vi "oa_Adjust DC Gap Data for Probe Orientation.vi"(6 "rotating settings":T1={"shaft rotating direction"=0, "probe orientation"={"X (red)"=0, "Y (blue)"=90}} {"shaft rotating direction" items=["CCW", "CW"]}, 8 "error in (no error)":errorcluster, 11 "DC Gap":cluster{"X":dbl[], "Y":dbl[]}[](array[cluster]) {"Y" format="%.2f"; "X" format="%.2f"}) -> (0 "error out":errorcluster, 3 "DC Gap out":cluster{"X":dbl[], "Y":dbl[]}[](array[cluster]) {"Y" format="%.2f"; "X" format="%.2f"})   [LabVIEW 2017]
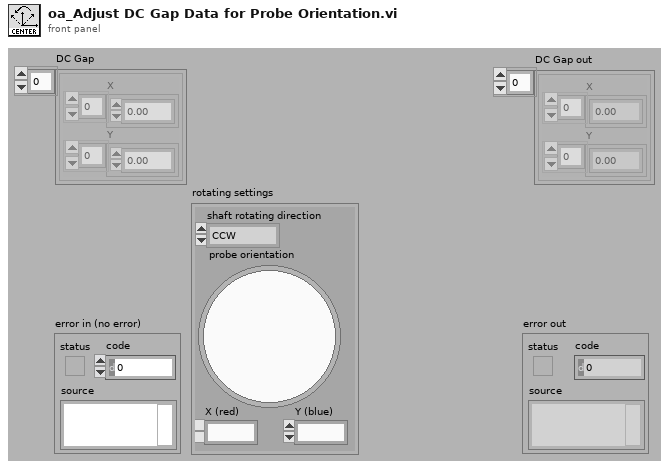
[diagram p1: front panel]
types:
  T1 = cluster{"shaft rotating direction":u16, "probe orientation":cluster{"X (red)":u32, "Y (blue)":u32}}
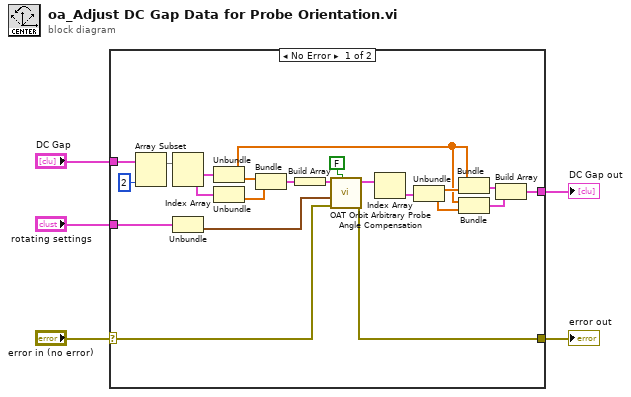
[diagram p0: block diagram]
diagram:
  n1 = case shown="No Error" "error in (no error)" {
    selector: "error in (no error)" -> [w25 w29]
    tunnel: [w23 w29] -> w4
    tunnel: "rotating settings" -> [w27 _]
    tunnel: [w6 w28] -> w2
    tunnel: "DC Gap" -> [w18 w28]
    frame No Error {
      n2 = Array Subset(array=w18, length=2) -> (w17:cluster{"X":dbl[], "Y":dbl[]}[])  [unwired: 1 in]
      n3 = Index Array(array=w17) -> (element #1=w22:cluster{"X":dbl[], "Y":dbl[]}, element #2=w21:cluster{"X":dbl[], "Y":dbl[]})  [unwired: 2 in]
      n4 = Unbundle(w27) -> ("probe orientation"=w26:cluster{"X (red)":u32, "Y (blue)":u32})  [unwired: 1 out]
      n5 = Unbundle(w22) -> ("X"=w10:dbl[], "Y"=w20:dbl[])
      n6 = Unbundle(w21) -> ("Y"=w19:dbl[])  [unwired: 1 out]
      n7 = Bundle("Y"=w20, "Y"=w19) -> (w15:cluster{"Y":dbl[], "Y":dbl[]})  [unwired: 1 in]
      n8 = Build Array(w15) -> (w14:cluster{"Y":dbl[], "Y":dbl[]}[])
      n9 = call <vilib>:"OAT Orbit Arbitrary Probe Angle Compensation.vi"("select methods"=FALSE, "error in (no error)"=w25, "probe angle"=w26, "XY plot data in"=w14) -> ("error out"=w23:errorcluster, "XY plot data out"=w13:cluster{dbl[], dbl[]}[])  [unwired: 5 in, 1 out]
      n10 = Index Array(array=w13) -> (element=w12:cluster{dbl[], dbl[]})  [unwired: 1 in]
      n11 = Unbundle(w12) -> (w11:dbl[], w9:dbl[])
      n12 = Bundle("X"=w10, w11) -> (w8:cluster{"X":dbl[], dbl[]})  [unwired: 1 in]
      n13 = Bundle("X"=w10, w9) -> (w7:cluster{"X":dbl[], dbl[]})  [unwired: 1 in]
      n14 = Build Array(w8, w7) -> (w6:cluster{"X":dbl[], dbl[]}[])
    }
    frame Error {
    }
  }
  "error out" <- w4
  "DC Gap out" <- w2
